vi "Format Tree.vi"(9 "Update":bool, 10 "Commands":cluster{"Time (s)":dbl, T1, bool}[](array[cluster]), 11 "Tree Refnum":refnum<vi>) -> ()   [LabVIEW 2019]
uses:
  Single Cmd Info.ctl
  <vilib>/picture/picture.llb/imagedata.ctl
  <vilib>/Utility/Data Type/NI_Data Type.lvlib
panel:
  in  "Tree":string(tree)
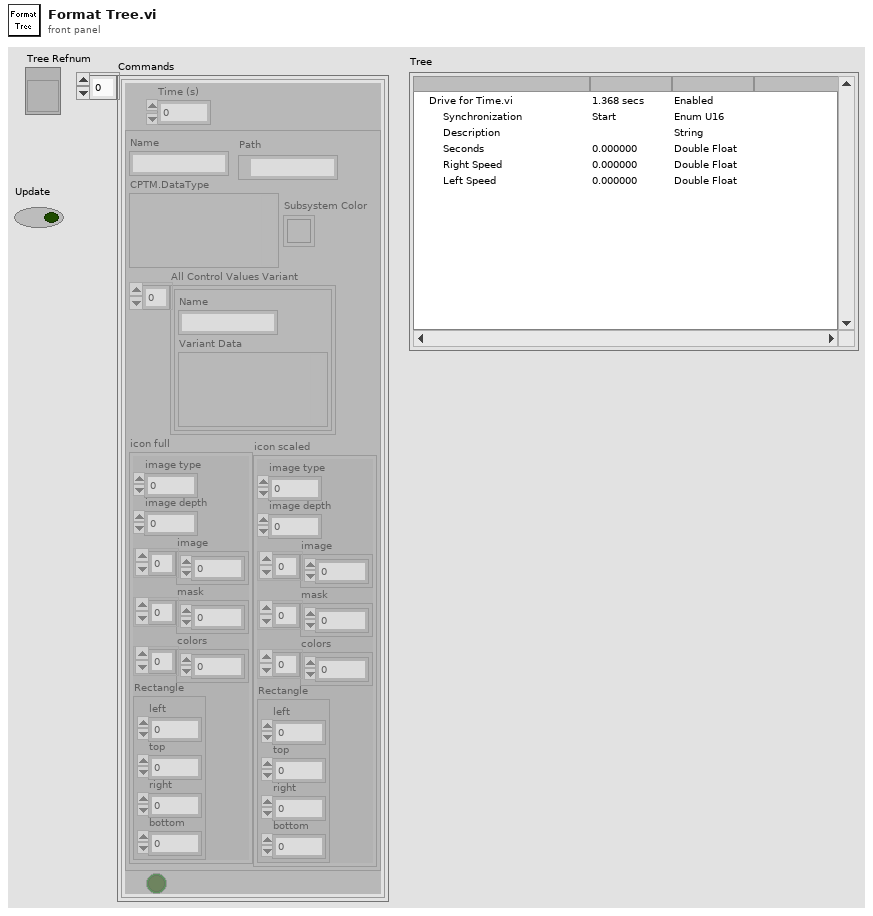
[diagram p1: front panel]
types:
  T1 = typedef "Single Cmd Info.ctl" = cluster{"Name":string, "CPTM.DataType":variant, "All Control Values Variant":cluster{"Name":string, "Variant Data":variant}[], "icon full":T2, "icon scaled":T2, "Path":path, "Subsystem Color":u32}
  T2 = typedef "imagedata.ctl" = cluster{"image type":i32, "image depth":i32, "image":u8[], "mask":u8[], "colors":u32[], "Rectangle":cluster{"left":i16, "top":i16, "right":i16, "bottom":i16}}
  T3 = cluster{"Left Cell String":string, "Child Text":string[], "Child Tag":string, "Item Indent":i32, "Child Only?":bool, "Glyph Index":i32}
  T4 = cluster{"Left Cell String":string, "Child Text":string[], "Child Tag":string, "Item Indent":i32, "Child Only?":bool, "Glyph Index":i32}[]
  T5 = typedef "NI_Data Type.lvlib/Data Type.ctl" = enum8{"Invalid Type", "Void", "I8", "I16", "I32", "I64", "U8", "U16", "U32", "U64", "Single Float", "Double Float", "Extended Float", "Single Complex", "Double Complex", "Extended Complex", "Enum U8", "Enum U16", "Enum U32", "Enum U64", "Single Float With Unit", "Double Float With Unit", "Extended Float With Unit", "Single Complex with Unit", "Double Complex with Unit", "Extended Complex with Unit", "Boolean", "String", "Path", "Picture", "Tag", "Array", "Cluster", "Variant", "LV Variant", "Waveform", "Timestamp", "Digital Waveform", "Digital Data", "ExpressData", "Refnum", "External Data", "VI", "Poly VI", "LabVIEW Class Instance", "Fixed Point", "Set Collection", "Map Collection"}
  T6 = typedef "NI_Data Type.lvlib/Type Definition Info.ctl" = cluster{"Name":string, "Timestamp":u32}
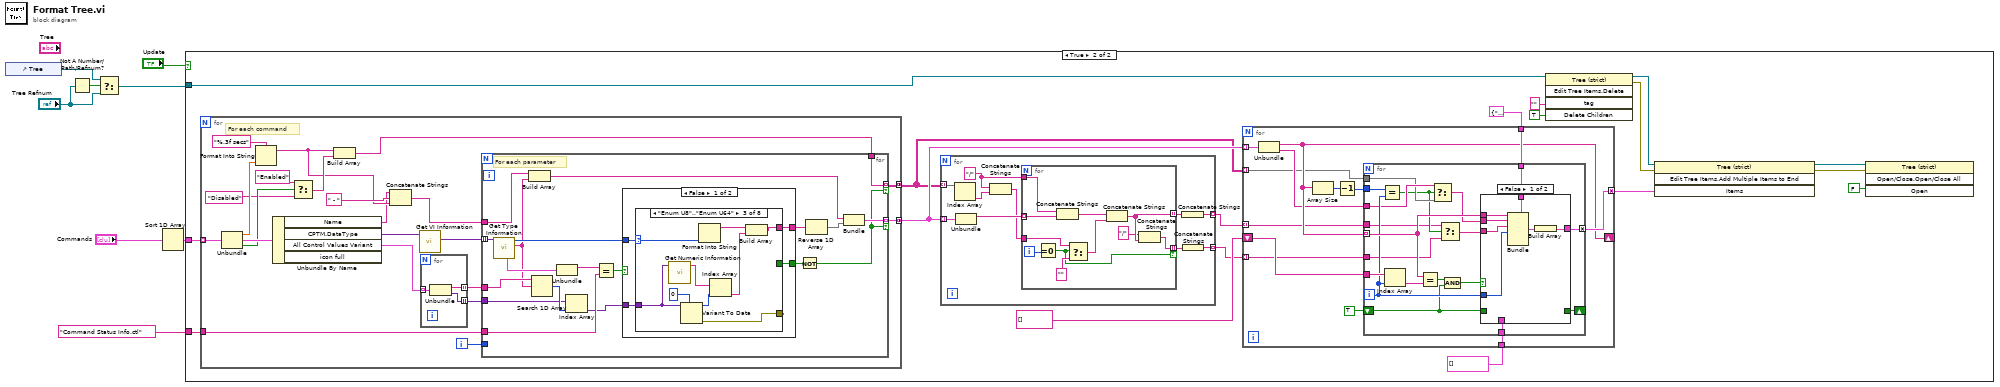
[diagram p0: block diagram]
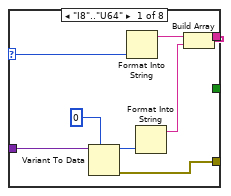
[diagram p4: hidden frame]
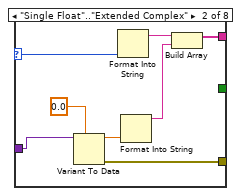
[diagram p5: hidden frame]
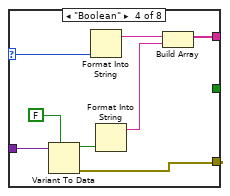
[diagram p6: hidden frame]
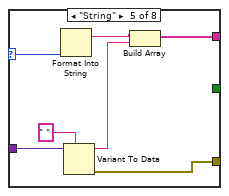
[diagram p7: hidden frame]
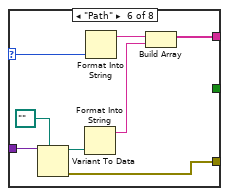
[diagram p8: hidden frame]
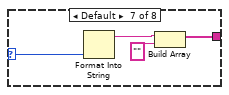
[diagram p9: hidden frame]
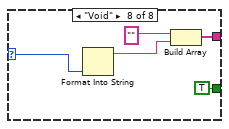
[diagram p10: hidden frame]
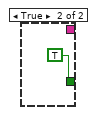
[diagram p11: hidden frame]
diagram:
  n1 = control-ref of="Tree"() -> (w6:refnum<vi>)
  n2 = Not A Number/Path/Refnum?(number/path/refnum="Tree Refnum") -> (NaN/Path/Refnum?=w8:bool)
  n3 = Select(t=w6, s=w8, f="Tree Refnum") -> (s? t:f=w3:refnum<vi>)
  n4 = Sort 1D Array(array="Commands") -> (sorted array=w2:cluster{"Time (s)":dbl, T1, bool}[])
  n5 = case shown="True" "Update" {
    tunnel: "Command Status Info.ctl" ("Name") -> [_ w26]
    tunnel: w3 -> [_ w13]
    tunnel: w2 -> [_ w12]
    frame False {
    }
    frame True {
      n6 = for {
        tunnel: [w87] -> w11 mode=concatenating
        tunnel: w26 -> [w82]
        tunnel: w12 -> [w80] mode=indexing
        tunnel: [w73] -> w10 mode=concatenating
        i -> [w83]
        # "For each command"
        n7 = Unbundle(w80) -> ("Time (s)"=w79:dbl, w81:T1, w78:bool)
        n8 = Format Into String(format string="%.3f secs", w79) -> (resulting string=w70:string)  [unwired: 2 in, 1 out]
        n9 = Unbundle By Name(w81) -> ("Name"=w69:string, "CPTM.DataType"=w89:variant, "All Control Values Variant"=w86:cluster{"Name":string, "Variant Data":variant}[])  [unwired: 1 out]
        n10 = Select(t="Enabled", s=w78, f="Disabled") -> (s? t:f=w75:string)
        n11 = Build Array(w70, w75) -> (w74:string[])
        n12 = Concatenate Strings(w69, " - ", w70) -> (w68:string)
        n13 = call <vilib>:"Get VI Information.vi"("variant"=w89) -> ("VI terminal types"=w88:variant[])  [unwired: 7 in, 3 out]
        n14 = for {
          tunnel: w86 -> [w173] mode=indexing
          tunnel: [w172] -> w85 mode=indexing
          tunnel: [w171] -> w84 mode=indexing
          n15 = Unbundle(w173) -> ("Name"=w172:string, "Variant Data"=w171:variant)
        }
        n16 = for {
          tunnel: w88 -> [w108] mode=indexing
          tunnel: [w105] -> w87 mode=indexing if=w90
          tunnel: w82 -> [w103]
          tunnel: w85 -> [w98]
          tunnel: w84 -> [w95]
          tunnel: w83 -> [_]
          tunnel: w68 -> [w93]
          tunnel: w74 -> [w91]
          tunnel: [w91] -> w73 mode=indexing if=w90
          # "For each parameter"
          n17 = call <vilib>:"Get Type Information.vi"("variant"=w108) -> ("name"=w97:string, "type"=w107:T5, "type definition info"=w104:T6)  [unwired: 6 in, 2 out]
          n18 = Build Array(w93, w97) -> (w106:string[])
          n19 = Search 1D Array(1D array=w98, element=w97) -> (index of element=w96:i32)  [unwired: 1 in]
          n20 = Unbundle(w104) -> ("Name"=w102:string)  [unwired: 1 out]
          n21 = Index Array(array=w95, index=w96) -> (element=w94:variant)
          n22 = Equal?(x=w102, y=w103) -> (x = y?=w101:bool)
          n23 = case shown="False" w101 {
            tunnel: w107 -> [w112 _]
            tunnel: [w111 _] -> w99
            tunnel: [w110 TRUE] -> w100
            tunnel: w94 -> [w109 _]
            frame False {
              n24 = case shown="\"Enum U8\"..\"Enum U64\"" w112 {
                selector: w112 -> [w120 w128 w137 w145 w152 w160 w164 w169]
                tunnel: [w115 w122 w134 w140 w149 w155 w162 w166] -> w111
                tunnel: [_ _ _ _ _ _ _ TRUE] -> w110
                tunnel: w109 -> [w114 w125 w132 w142 w151 w157 _ _]
                tunnel: [w113 w121 w133 w138 w146 w153 _ _] -> _
                frame "I8".."U64" {
                  n25 = Variant To Data(type=i64 0, Variant=w114) -> (data=w118:i64, error out=w113:errorcluster)  [unwired: 1 in]
                  n26 = Format Into String(w120) -> (resulting string=w116:string)  [unwired: 3 in, 1 out]
                  n27 = Format Into String(w118) -> (resulting string=w117:string)  [unwired: 3 in, 1 out]
                  n28 = Build Array(w116, w117) -> (w115:string[])
                }
                frame "Single Float".."Extended Complex" {
                  n29 = Variant To Data(type=0.0, Variant=w125) -> (data=w126:dbl, error out=w121:errorcluster)  [unwired: 1 in]
                  n30 = Format Into String(w128) -> (resulting string=w124:string)  [unwired: 3 in, 1 out]
                  n31 = Format Into String(w126) -> (resulting string=w123:string)  [unwired: 3 in, 1 out]
                  n32 = Build Array(w124, w123) -> (w122:string[])
                }
                frame "Enum U8".."Enum U64" {
                  n33 = call <vilib>:"Get Numeric Information.vi"("variant"=w132) -> ("enum names"=w131:string[])  [unwired: 7 in, 3 out]
                  n34 = Variant To Data(type=i64 0, Variant=w132) -> (data=w130:i64, error out=w133:errorcluster)  [unwired: 1 in]
                  n35 = Format Into String(w137) -> (resulting string=w135:string)  [unwired: 3 in, 1 out]
                  n36 = Index Array(array=w131, index=w130) -> (element=w129:string)
                  n37 = Build Array(w135, w129) -> (w134:string[])
                }
                frame "Boolean" {
                  n38 = Variant To Data(type=FALSE, Variant=w142) -> (data=w143:bool, error out=w138:errorcluster)  [unwired: 1 in]
                  n39 = Format Into String(w145) -> (resulting string=w141:string)  [unwired: 3 in, 1 out]
                  n40 = Format Into String(w143) -> (resulting string=w139:string)  [unwired: 3 in, 1 out]
                  n41 = Build Array(w141, w139) -> (w140:string[])
                }
                frame "String" {
                  n42 = Format Into String(w152) -> (resulting string=w150:string)  [unwired: 3 in, 1 out]
                  n43 = Variant To Data(type=" ", Variant=w151) -> (data=w148:string, error out=w146:errorcluster)  [unwired: 1 in]
                  n44 = Build Array(w150, w148) -> (w149:string[])
                }
                frame "Path" {
                  n45 = Variant To Data(type=path "", Variant=w157) -> (data=w158:path, error out=w153:errorcluster)  [unwired: 1 in]
                  n46 = Format Into String(w158) -> (resulting string=w154:string)  [unwired: 3 in, 1 out]
                  n47 = Format Into String(w160) -> (resulting string=w156:string)  [unwired: 3 in, 1 out]
                  n48 = Build Array(w156, w154) -> (w155:string[])
                }
                frame Default {
                  n49 = Format Into String(w164) -> (resulting string=w163:string)  [unwired: 3 in, 1 out]
                  n50 = Build Array(w163, "") -> (w162:string[])
                }
                frame "Void" {
                  n51 = Format Into String(w169) -> (resulting string=w167:string)  [unwired: 3 in, 1 out]
                  n52 = Build Array("", w167) -> (w166:string[])
                }
              }
            }
            frame True {
            }
          }
          n53 = Not(x=w100) -> (.not. x?=w90:bool)
          n54 = Reverse 1D Array(array=w99) -> (reversed array=w92:string[])
          n55 = Bundle(w106, w92) -> (w105:cluster{string[], string[]})  [unwired: 1 in]
        }
      }
      n56 = for {
        tunnel: w11 -> [w183] mode=indexing
        tunnel: [w180] -> w23 mode=indexing
        tunnel: w10 -> [w179] mode=indexing
        tunnel: [w175] -> w9 mode=indexing
        w174 = "/"
        n57 = Index Array(array=w179) -> (element=w178:string)  [unwired: 1 in]
        n58 = Unbundle(w183) -> (w182:string[])  [unwired: 1 out]
        n59 = Concatenate Strings(w174, w178) -> (w177:string)
        n60 = for {
          tunnel: w182 -> [w194] mode=indexing
          tunnel: [w187] -> w181 mode=indexing
          tunnel: w177 -> [w190]
          tunnel: [w186] -> w176 mode=indexing if=w188
          tunnel: w174 -> [w184]
          i -> [w193]
          n61 = Equal To 0?(x=w193) -> (x = 0?=w188:bool)
          n62 = Concatenate Strings(w184, w194) -> (w192:string)
          n63 = Select(t=w190, s=w188, f="") -> (s? t:f=w189:string)
          n64 = Concatenate Strings(w192, w189) -> (w187:string)
          n65 = Concatenate Strings("/", w187) -> (w186:string)
        }
        n66 = Concatenate Strings(w181) -> (w180:string)
        n67 = Concatenate Strings(w176) -> (w175:string)
      }
      n68 = for {
        tunnel: [w35] -> w14 mode=concatenating
        tunnel: T3 {"Left Cell String"="", "Child Text"=[], "Child Tag"="", "Item Indent"=0, "Child Only?"=FALSE, "Glyph Index"=0} ("Item") -> [w36]
        shift-right: [w32] -> _
        shift-left: string[] [] ("Child Text") -> [w38]
        tunnel: w11 -> [w39] mode=indexing
        tunnel: T4 [] -> [w37]
        tunnel: w23 -> [w31] mode=indexing
        tunnel: w10 -> [w28] mode=indexing
        tunnel: w9 -> [w27] mode=indexing
        n69 = Unbundle(w39) -> (w32:string[], w29:string[])
        n70 = Array Size(array=w32) -> (size(s)=w34:i32)
        n71 = Decrement(x=w34) -> (x-1=w33:i32)
        n72 = for {
          tunnel: w38 -> [w58]
          tunnel: w32 -> [w53] mode=indexing
          tunnel: w37 -> [w56]
          tunnel: [w55] -> w35 mode=concatenating
          tunnel: w36 -> [w54]
          tunnel: w33 -> [w51]
          tunnel: w29 -> [w45]
          tunnel: w31 -> [w41]
          shift-right: [w48] -> _
          shift-left: TRUE -> [w47]
          tunnel: w28 -> [w44]
          tunnel: w27 -> [w40]
          i -> [w52]
          n73 = Equal?(x=w51, y=w52) -> (x = y?=w43:bool)
          n74 = Index Array(array=w58, index=w52) -> (element=w57:string)
          n75 = Equal?(x=w53, y=w57) -> (x = y?=w50:bool)
          n76 = Select(t=w45, s=w43, f=w44) -> (s? t:f=w46:string[])
          n77 = Select(t=w41, s=w43, f=w40) -> (s? t:f=w42:string)
          n78 = And(x=w50, y=w47) -> (x .and. y?=w49:bool)
          n79 = case shown="False" w49 {
            tunnel: [w63 w67] -> w55
            tunnel: w56 -> [_ w67]
            tunnel: w54 -> [w65 _]
            tunnel: w53 -> [w62 _]
            tunnel: w52 -> [w61 _]
            tunnel: w46 -> [w60 _]
            tunnel: w42 -> [w59 _]
            tunnel: [_ w66] -> w48
            tunnel: w47 -> [_ w66]
            frame False {
              n80 = Bundle(cluster=w65, "Left Cell String"=w62, "Child Text"=w60, "Child Tag"=w59, "Item Indent"=w61) -> (w64:T3)  [unwired: 2 in]
              n81 = Build Array(w64) -> (w63:T4)
            }
            frame True {
            }
          }
        }
      }
      n82 = invoke on="Invoke Node" class="Tree (strict)" method="Edit Tree Items.Delete"(reference=w13, "tag"="" ("Tag"), "Delete Children"=TRUE ("Delete Children?")) -> (reference out=w20:refnum<vi>, error out=w15:errorcluster)  [unwired: 2 in, 3 out]
      n83 = invoke on="Invoke Node" class="Tree (strict)" method="Edit Tree Items.Add Multiple Items to End"(reference=w20, error in=w15, "Items"=w14) -> (reference out=w21:refnum<vi>, error out=w18:errorcluster)  [unwired: 1 in, 2 out]
      n84 = invoke on="Invoke Node" class="Tree (strict)" method="Open/Close.Open/Close All"(reference=w21, error in=w18, "Open"=FALSE ("Open?")) -> ()  [unwired: 1 in, 4 out]
    }
  }
